vi "Host Main.vi"() -> ()   [LabVIEW 2014]
doc: "This application launches and executes the Tag Bus Data framework configuration for the specified target alias. This is a simple example of the framework API functions, but may also be a suitable starting point for a Host UI or Thick Client that is running a local version of the framework."
uses:
  <vilib>/NI/Module Execution Interface/Engine Runtime/Execution States.ctl
  <vilib>/NI/Module Execution Interface/Engine Runtime/Fault.ctl
  <vilib>/NI/Tag Bus Module Framework/runtime/error classification.ctl
  <vilib>/NI/Module Execution Interface/Engine Runtime/Engine Runtime Interface.lvclass
  <vilib>/NI/DCAF/Tag Editor Core/Framework Configuration Classes/target runtime/PL_Target Runtime.lvclass
  <vilib>/NI/Tag Bus Module Framework/runtime/TBM module execution interface.lvclass
panel:
  in  "Error3":bool
  in  "Error2":bool
  in  "Error1":bool
  in  "target alias":string="PC"
  out "engine status":T4(array[cluster])
  in  "stop":bool
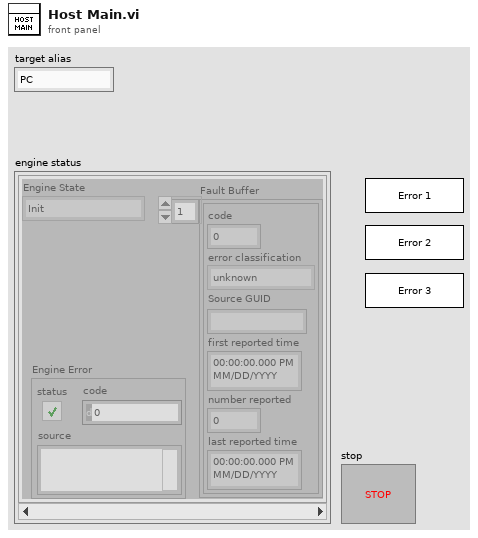
[diagram p1: front panel]
types:
  T1 = typedef "Engine Runtime Interface.lvclass/Execution States.ctl" = enum16{"Init", "Pre-Operational", "Safe-Operational", "Operational", "Stopped"}
  T2 = typedef "Engine Runtime Interface.lvclass/Fault.ctl" = cluster{"code":i32, "error classification":T3, "Source GUID":string, "first reported time":timestamp, "number reported":u32, "last reported time":timestamp}
  T3 = typedef "TBM module execution interface.lvclass/error classification.ctl" = enum16{"unknown", "none", "trivial", "recoverable", "critical"}
  T4 = cluster{"Engine State":T1, "Fault Buffer":T2[], "Engine Error":errorcluster}[]
  T5 = cluster{"Engine State":T1, "faults":T2[], "Engine Error":errorcluster}
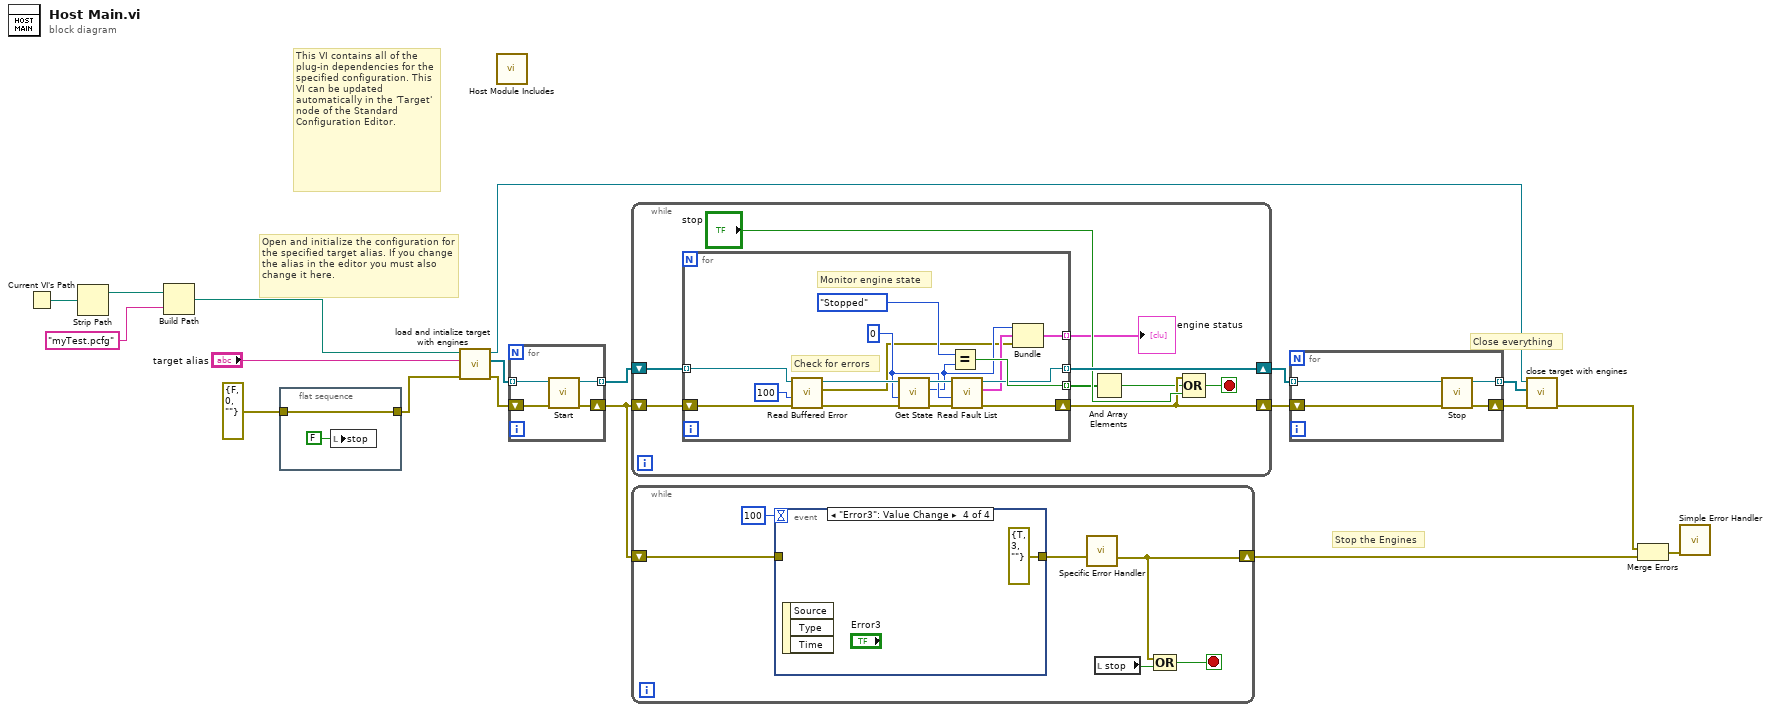
[diagram p0: block diagram]
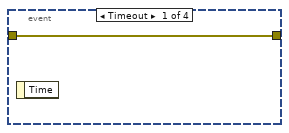
[diagram p2: hidden frame]
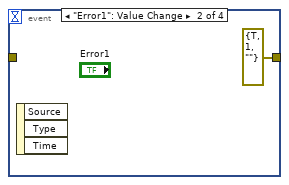
[diagram p3: hidden frame]
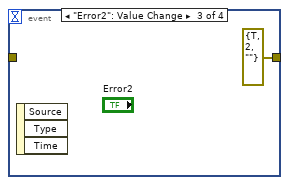
[diagram p4: hidden frame]
diagram:
  # "Open and initialize the configuration for the specified target alias. If you change the alias in the editor you must also change it here."
  # "Close everything"
  # "Stop the Engines"
  # "This VI contains all of the plug-in dependencies for the specified configuration. This VI can be updated automatically in the 'Target' node of the Standard Configuration Editor."
  n1 = Current VI's Path() -> (path=w7:path)
  n2 = Strip Path(path=w7) -> (stripped path=w6:path)  [unwired: 1 out]
  n3 = Build Path(base path=w6, name or relative path="myTest.pcfg") -> (appended path=w4:path)
  n4 = flat-sequence {
    tunnel: errorcluster {"status"=FALSE, "code"=0, "source"=""} ("error in") -> [w20]
    tunnel: [w20] -> w2
    frame #0 {
      n5 = local write "stop"(FALSE ("stop")) -> ()
    }
  }
  n6 = call <vilib>:"load and intialize target with engines.vi"("error in"=w2, "target alias"="target alias", "file path"=w4) -> ("error out"=w16:errorcluster, "engine runtime interfaces"=w15:refnum<class "Engine Runtime Interface.lvclass">[], "target runtime"=w12:refnum<class "PL_Target Runtime.lvclass">)  [unwired: 6 in]
  n7 = call "Host Module Includes.vi"() -> ()  [unwired: 12 in]
  n8 = for {
    tunnel: [w25] -> w19 mode=indexing
    tunnel: w15 -> [w22] mode=indexing
    shift-right: [w24] -> w10
    shift-left: w16 -> [w23]
    n9 = call-dynamic "Start.vi"("error in"=w23, "Engine Runtime Interface in"=w22) -> ("error out"=w24:errorcluster, "Engine Runtime Interface out"=w25:refnum<class "Engine Runtime Interface.lvclass">)  [unwired: 8 in]
  }
  n10 = while {
    shift-right: [w32] -> w18
    shift-left: w19 -> [w34]
    shift-right: [w29] -> w17
    shift-left: w10 -> [w33]
    stop <- w30 stop-if-true
    n11 = for {
      tunnel: w34 -> [w50] mode=indexing
      tunnel: [w41] -> w32 mode=indexing
      tunnel: [w45] -> w27 mode=indexing
      shift-right: [w40] -> w29
      shift-left: w33 -> [w49]
      tunnel: [w35] -> w28 mode=indexing
      w39 = 0 ("timeout (-1)")
      # "Monitor engine state"
      # "Check for errors"
      n12 = call-dynamic "Read Buffered Error.vi"("error in"=w49, "timeout in ms (0)"=100, "Engine Runtime Interface in"=w50) -> ("error out"=w47:errorcluster, "Engine Error"=w36:errorcluster, "Engine Runtime Interface out"=w48:refnum<class "Engine Runtime Interface.lvclass">)  [unwired: 6 in]
      n13 = call-dynamic "Get State.vi"("error in"=w47, "timeout (-1)"=w39, "Engine Runtime Interface in"=w48) -> ("error out"=w43:errorcluster, "Engine State"=w38:T1, "Engine Runtime Interface out"=w42:refnum<class "Engine Runtime Interface.lvclass">)  [unwired: 6 in]
      n14 = Equal?(x=Execution_States."Stopped" ("Engine State"), y=w38) -> (x = y?=w45:bool)
      n15 = call-dynamic "Read Fault List.vi"("error in"=w43, "timeout (-1)"=w39, "Engine Runtime Interface in"=w42) -> ("error out"=w40:errorcluster, "faults"=w37:T2[], "Engine Runtime Interface out"=w41:refnum<class "Engine Runtime Interface.lvclass">)  [unwired: 6 in]
      n16 = Bundle("Engine State"=w38, "faults"=w37, "Engine Error"=w36) -> (w35:T5)  [unwired: 1 in]
    }
    "engine status" <- w28
    n17 = And Array Elements(Boolean array=w27) -> (logical AND=w26:bool)
    n18 = Compound Arithmetic op=OR(w29, w26, "stop") -> (w30:bool)
  }
  n19 = while {
    shift-right: [w52] -> w9
    shift-left: w10 -> [w55]
    stop <- w51 stop-if-true
    n20 = event shown="[3] \"Error3\": Value Change" {
      selector: _ -> [_ _ _ _]
      dyn-events: _ -> [_ _ _ _]
      timeout: 100 -> [_ _ _ _]
      tunnel: w55 -> [w57 _ _ _]
      tunnel: [w57 errorcluster {"status"=TRUE, "code"=1, "source"=""} ("error out") errorcluster {"status"=TRUE, "code"=2, "source"=""} ("error out") errorcluster {"status"=TRUE, "code"=3, "source"=""} ("error out")] -> w54
      event Timeout {
        n21 = event-data() -> ()  [unwired: 1 in, 1 out]
      }
      event "Error1": Value Change {
        n22 = event-data() -> ()  [unwired: 1 in, 3 out]
      }
      event "Error2": Value Change {
        n23 = event-data() -> ()  [unwired: 1 in, 3 out]
      }
      event "Error3": Value Change {
        n24 = event-data() -> ()  [unwired: 1 in, 3 out]
      }
    }
    n25 = call "Specific Error Handler"("Error to Check"=w54) -> ("error out"=w52:errorcluster)  [unwired: 11 in, 3 out]
    n26 = local read "stop"() -> (w53:bool)
    n27 = Compound Arithmetic op=OR(w52, w53) -> (w51:bool)
  }
  n28 = for {
    tunnel: w18 -> [w64] mode=indexing
    shift-right: [w61] -> w11
    shift-left: w17 -> [w63]
    tunnel: [w62] -> w13 mode=indexing
    n29 = call-dynamic "Stop.vi"("error in"=w63, "Engine Runtime Interface in"=w64) -> ("error out"=w61:errorcluster, "Engine Runtime Interface out"=w62:refnum<class "Engine Runtime Interface.lvclass">)  [unwired: 8 in]
  }
  n30 = call <vilib>:"close target with engines.vi"("error in"=w11, "Engine Runtime Interfaces"=w13, "Target Runtime"=w12) -> ("error out"=w1:errorcluster)  [unwired: 8 in]
  n31 = Merge Errors(w1, w9) -> (w8:errorcluster)
  n32 = call <vilib>:"Simple Error Handler.vi"("error in (no error)"=w8) -> ()  [unwired: 4 in, 5 out]
